vi "RVTBOX SampleCode.vi"(11 "Modbus TCP Setting":T1={"TCP address"="192.168.1.38", "CH"=enum."Port1", "Sample Rate"=7812, "Port"=502}) -> ()   [LabVIEW 2022 SP3]
uses:
  Ctl/Modbus Function TCP.ctl
  Ctl/TCP Setting.ctl
  DLL/Modbus.dll
panel:
  out "Waveform Chart":dbl[][](graph)=[[0.0015869140625, -0.000732421875, -0.001220703125], [0.0008544921875, -0.0009765625, 0.000244140625], [0.0006103515625, -0.001220703125, 0.001220703125], [0.0015869140625, -0.0006103515625, 0.00048828125], [0.001953125, 0.0, -0.00048828125], [0.0009765625, 0.0, -0.000732421875], [0.0010986328125, -0.000244140625, -0.0006103515625], [0.0020751953125, 0.000244140625, 0.0], [0.002197265625, 0.001220703125, 0.0006103515625], [0.0020751953125, 0.0009765625, -0.000244140625], [0.0020751953125, 0.0, -0.0018310546875], [0.0013427734375, 0.0, -0.001708984375], [0.00048828125, 0.0001220703125, -0.0008544921875], [0.0009765625, -0.000244140625, -0.0010986328125], [0.0009765625, -0.0008544921875, -0.00146484375], [-0.0003662109375, -0.0003662109375, -0.0003662109375], [-0.0010986328125, 0.0, 0.0001220703125], [-0.0003662109375, -0.000244140625, -0.0008544921875], [-0.0006103515625, -0.000244140625, -0.001708984375], [-0.00146484375, 0.0010986328125, 0.0], [-0.000732421875, 0.001953125, 0.002685546875], [0.000244140625, 0.0010986328125, 0.0037841796875], [0.0, 0.0003662109375, 0.002197265625], [-0.0006103515625, 0.0006103515625, -0.0006103515625]]
  out "Modbus Function":T2
  out "Failure  (Port1 ~ Port4)":bool[](array[boolean])
  out "Connted (Port1 ~ Port4)":bool[](array[boolean])
  out "Device ID":u16
  out "Stop Time":timestamp
  in  "stop":bool
  out "Data Length 抓資料後的剩餘長度":u16(graph)
  out "Iteration":i32
  out "Next #":u16
  out "error out":errorcluster
  # "BOX只能一次抓一個PORT 無法同時抓4個"
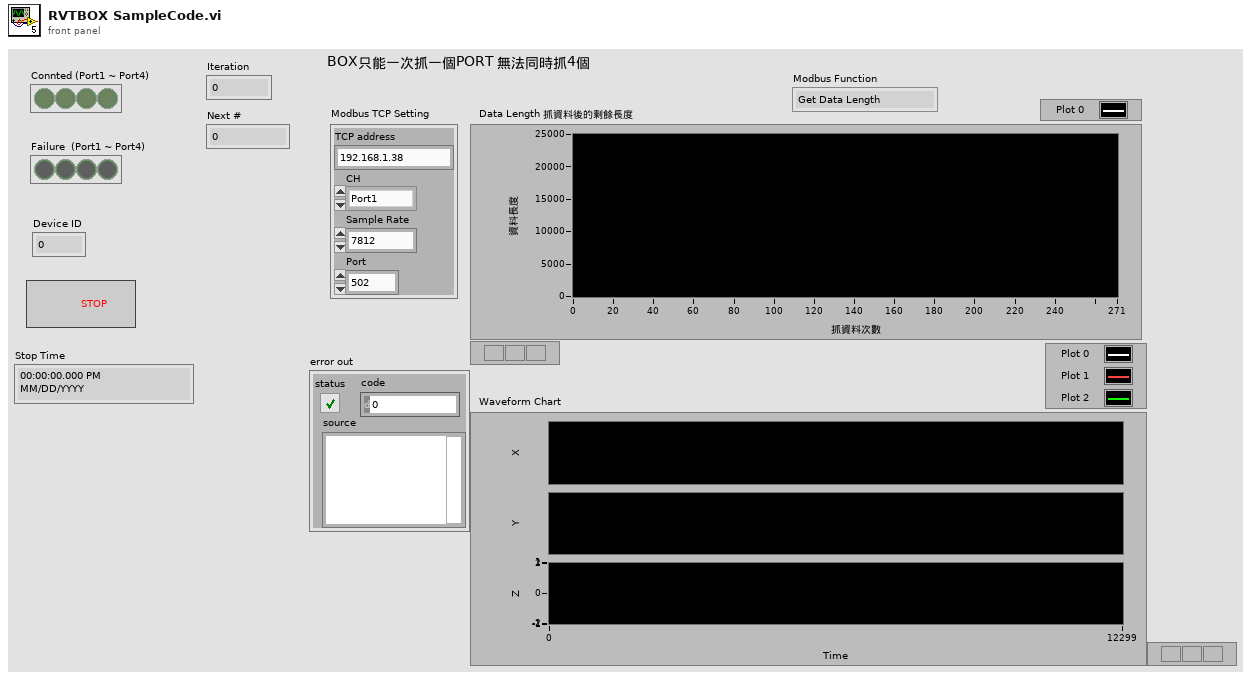
[diagram p1: front panel]
types:
  T1 = typedef "TCP Setting.ctl" = cluster{"TCP address":string, "CH":enum16{"Port1", "Port2", "Port3", "Port4"}, "Sample Rate":u16, "Port":i32}
  T2 = typedef "Modbus Function TCP.ctl" = enum16{"Get Data Length", "Normal Mode", "Bulk Mode", "Reconnect Port", "Recconect Box"}
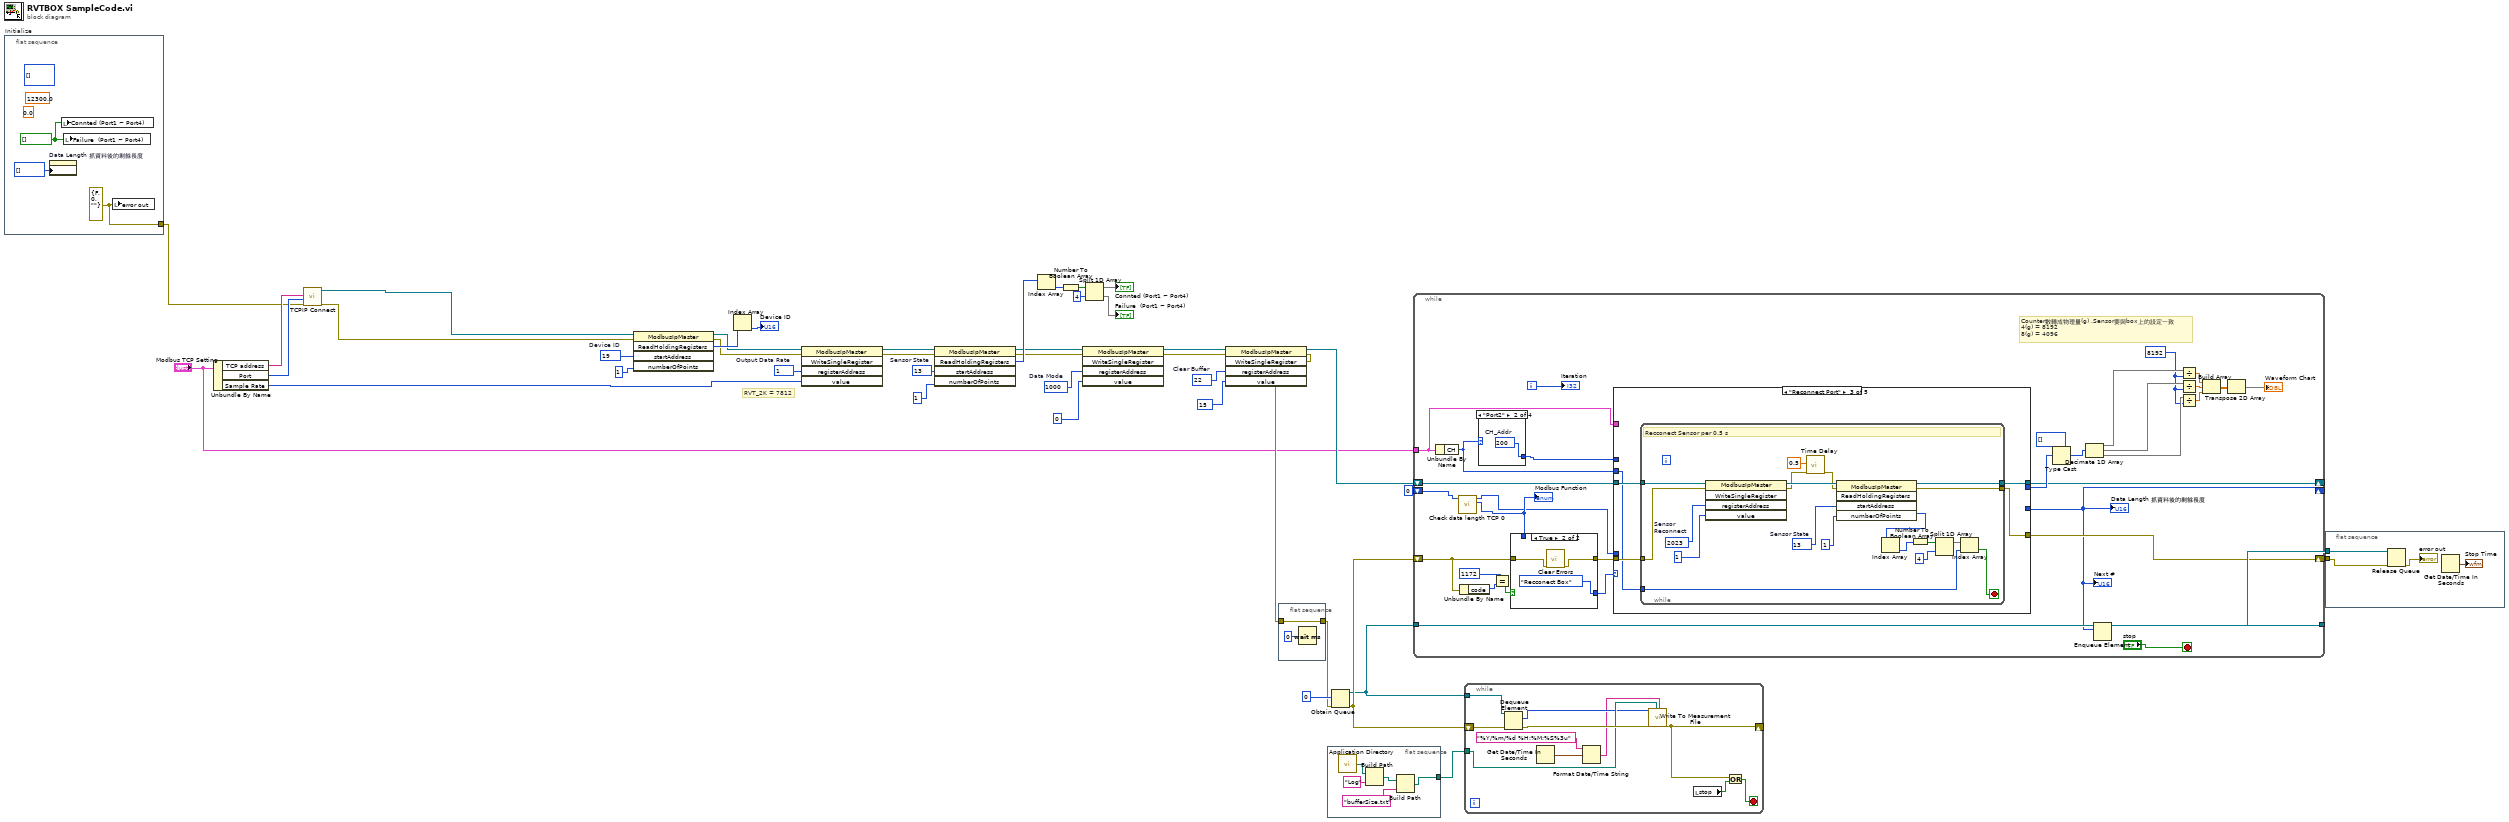
[diagram p0: block diagram]
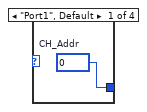
[diagram p3: hidden frame]
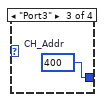
[diagram p4: hidden frame]
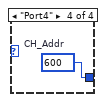
[diagram p5: hidden frame]
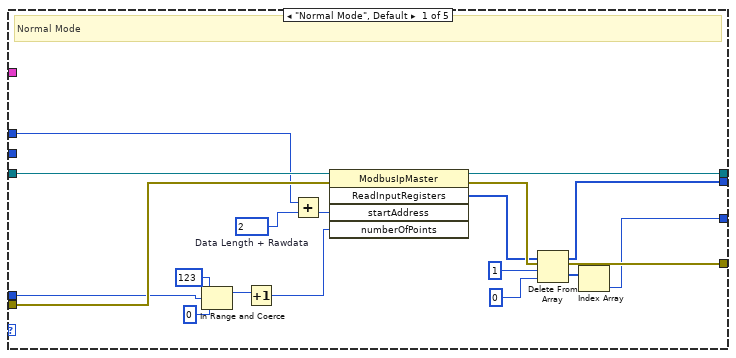
[diagram p6: hidden frame]
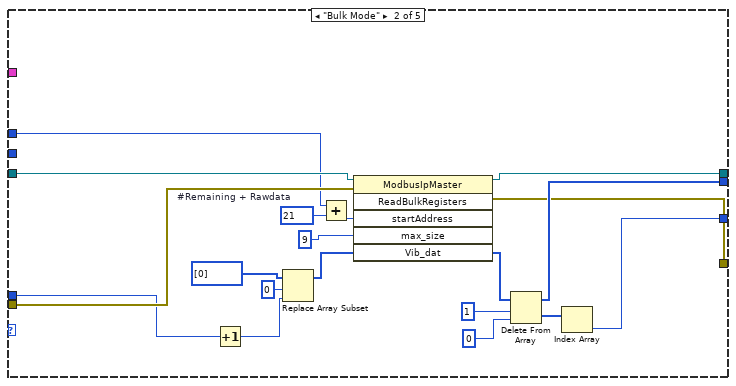
[diagram p7: hidden frame]
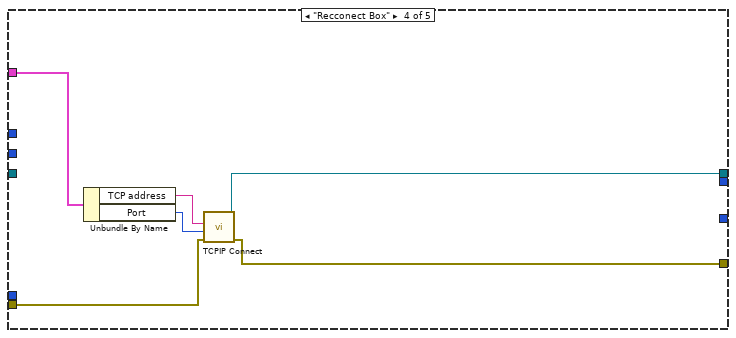
[diagram p8: hidden frame]
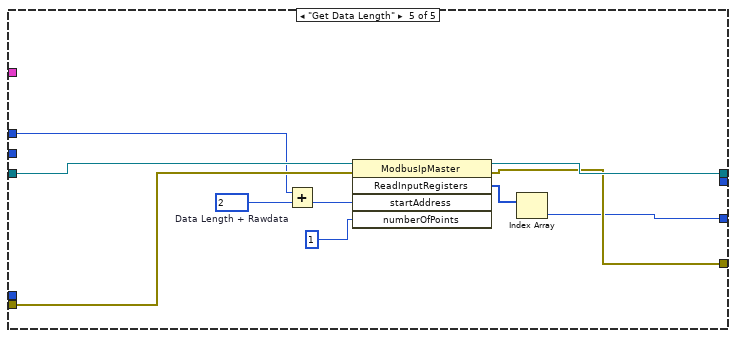
[diagram p9: hidden frame]
diagram:
  w14 = u16 1000  # Data Mode
  w17 = u16 22  # Clear Buffer
  w27 = u16 13  # Sensor State
  w32 = u16 19  # Device ID
  w34 = u16 1  # Output Data Rate
  # "RVT_2K = 7812"
  n1 = flat-sequence "Initialize" {
    tunnel: [w45] -> w7
    frame #0 {
      (unwired) 12300.0 ("X Scale.Range:Maximum")
      (unwired) 0.0 ("X Scale.Range:Minimum")
      (unwired) i16[][] []
      w44 = bool[] [] ("Failure ? (Port1 ~ Port4)")
      w45 = errorcluster {"status"=FALSE, "code"=0, "source"=""} ("error out")
      n2 = property on="Data Length 抓資料後的剩餘長度" class="WFChart (strict)"("History Data"=u16[] []) -> ()  [unwired: 2 in, 2 out]
      n3 = local write "Connted (Port1 ~ Port4)"(w44) -> ()
      n4 = local write "Failure  (Port1 ~ Port4)"(w44) -> ()
      n5 = local write "error out"(w45) -> ()
    }
  }
  n6 = Unbundle By Name("Modbus TCP Setting") -> ("TCP address"=w9:string, "Port"=w8:i32, "Sample Rate"=w11:u16)
  n7 = call "TCPIP Connect.vi"("error in (no error)"=w7, "Port"=w8, "TCP address"=w9) -> ("error out"=w1:errorcluster, "CreateIp"=w2:refnum<k24>)  [unwired: 7 in]
  n8 = invoke class="ModbusIpMaster" method="ReadHoldingRegisters"(reference=w2, error in=w1, "startAddress"=w32, "numberOfPoints"=u16 1) -> (reference out=w4:refnum<k24>, error out=w3:errorcluster, "ReadHoldingRegisters"=w31:u16[])  [unwired: 1 in, 2 out]
  n9 = Index Array(array=w31) -> (element=→"Device ID":u16)  [unwired: 1 in]
  n10 = invoke class="ModbusIpMaster" method="WriteSingleRegister"(reference=w4, error in=w3, "registerAddress"=w34, "value"=w11) -> (reference out=w25:refnum<k24>, error out=w24:errorcluster)  [unwired: 1 in, 3 out]
  n11 = invoke class="ModbusIpMaster" method="ReadHoldingRegisters"(reference=w25, error in=w24, "startAddress"=w27, "numberOfPoints"=u16 1) -> (reference out=w6:refnum<k24>, error out=w5:errorcluster, "ReadHoldingRegisters"=w23:u16[])  [unwired: 1 in, 2 out]
  n12 = Index Array(array=w23) -> (element=w22:u16)  [unwired: 1 in]
  n13 = Number To Boolean Array(number=w22) -> (Boolean array=w20:bool[])
  n14 = invoke class="ModbusIpMaster" method="WriteSingleRegister"(reference=w6, error in=w5, "registerAddress"=w14, "value"=u16 0) -> (reference out=w13:refnum<k24>, error out=w12:errorcluster)  [unwired: 1 in, 3 out]
  n15 = Split 1D Array(array=w20, index=4) -> (first subarray=→"Connted (Port1 ~ Port4)":bool[], second subarray=→"Failure  (Port1 ~ Port4)":bool[])
  n16 = invoke class="ModbusIpMaster" method="WriteSingleRegister"(reference=w13, error in=w12, "registerAddress"=w17, "value"=u16 15) -> (reference out=w28:refnum<k24>, error out=w29:errorcluster)  [unwired: 1 in, 3 out]
  n17 = flat-sequence {
    tunnel: w29 -> [w46]
    tunnel: [w46] -> w39
    frame #0 {
      n18 = Wait (ms)(milliseconds to wait=u32 0) -> ()  [unwired: 1 out]
    }
  }
  n19 = flat-sequence {
    tunnel: [w48] -> w35
    frame #0 {
      n20 = call <vilib>:"Application Directory.vi"() -> ("Application Directory"=w52:path)
      n21 = Build Path(base path=w52, name or relative path="Log") -> (appended path=w50:path)
      n22 = Build Path(base path=w50, name or relative path="bufferSize.txt") -> (appended path=w48:path)
    }
  }
  n23 = Obtain Queue(element data type=u16 0 ("Next # 2"), error in (no error)=w39) -> (queue out=w37:refnum<queue>, error out=w38:errorcluster)  [unwired: 3 in, 1 out]
  n24 = while {
    shift-right: [w79] -> w42
    shift-left: w38 -> [w68]
    shift-right: [w77] -> _
    shift-left: u16 0 ("# samples in buffer") -> [w64]
    shift-right: [w75] -> _
    shift-left: w28 -> [w84]
    tunnel: w37 -> [w78]
    tunnel: [w76] -> w36
    tunnel: "Modbus TCP Setting" -> [w65]
    i -> [w83]
    stop <- "stop" stop-if-true
    w58 = 8192 ("length")
    # "Counter數轉成物理量(g) ,Sensor要與box上的設定一致\n4(g) = 8192\n8(g) = 4096"
    n25 = Unbundle By Name(w65) -> ("CH"=w66:enum16{"Port1", "Port2", "Port3", "Port4"})
    n26 = call "Check data length TCP 0.vi"("# samples in buffer"=w64) -> ("Modbus Function"=w63:T2, "# samples in buffer out"=w62:u16)  [unwired: 9 in]
    "Modbus Function" <- w63
    n27 = Unbundle By Name(w68) -> ("code"=w72:i32)
    n28 = case shown="\"Port2\"" w66 {
      tunnel: [w90 w91 w92 w93] -> w74
      frame "Port1", Default {
        w90 = u16 0  # CH_Addr
      }
      frame "Port2" {
        w91 = u16 200  # CH_Addr
      }
      frame "Port3" {
        w92 = u16 400  # CH_Addr
      }
      frame "Port4" {
        w93 = u16 600  # CH_Addr
      }
    }
    n29 = Equal?(x=1172, y=w72) -> (x = y?=w70:bool)
    n30 = case shown="True" w70 {
      tunnel: [w85 Modbus_Function_TCP."Recconect Box" ("Modbus Function 2")] -> w69
      tunnel: w68 -> [w86 w89]
      tunnel: [w86 w88] -> w67
      tunnel: w63 -> [w85 _]
      frame False {
      }
      frame True {
        n31 = call <vilib>:"Clear Errors.vi"("error in (no error)"=w89) -> ("error out"=w88:errorcluster)  [unwired: 5 in, 1 out]
      }
    }
    n32 = case shown="\"Reconnect Port\"" w69 {
      tunnel: w84 -> [w99 w116 w135 _ w168]
      tunnel: [w101 w120 _ _ w164] -> w77
      tunnel: [w103 w118 w132 w156 w166] -> w79
      tunnel: [w100 w115 w131 w155 w167] -> w75
      tunnel: w67 -> [w104 w117 w134 w157 w169]
      tunnel: [w102 w119 _ _ _] -> w81
      tunnel: w62 -> [w96 w114 _ _ _]
      tunnel: w74 -> [w94 w112 _ _ w161]
      tunnel: w66 -> [_ _ w133 _ _]
      tunnel: w65 -> [_ _ _ w160 _]
      frame "Normal Mode", Default {
        w109 = u16 2  # Data Length + Rawdata
        # "Normal Mode"
        n33 = In Range and Coerce(upper limit=u16 123, x=w96, lower limit=u16 0) -> (coerced(x)=w105:u16)  [unwired: 1 out]
        n34 = Increment(x=w105) -> (x+1=w98:u16)
        n35 = Add(x=w94, y=w109) -> (x+y=w95:u16)
        n36 = invoke class="ModbusIpMaster" method="ReadInputRegisters"(reference=w99, error in=w104, "startAddress"=w95, "numberOfPoints"=w98) -> (reference out=w100:refnum<k24>, error out=w103:errorcluster, "ReadInputRegisters"=w97:u16[])  [unwired: 1 in, 2 out]
        n37 = Delete From Array(array=w97, length=1, index=0) -> (deleted portion=w108:u16[], array with subset deleted=w102:u16[])
        n38 = Index Array(array=w108) -> (element=w101:u16)  [unwired: 1 in]
      }
      frame "Bulk Mode" {
        w129 = u16 21  # #Remaining + Rawdata
        n39 = Increment(x=w114) -> (x+1=w123:u16)
        n40 = Replace Array Subset(array=u16[] [0], new element=w123, index=0) -> (w127:u16[])
        n41 = Add(x=w112, y=w129) -> (x+y=w113:u16)
        n42 = invoke class="ModbusIpMaster" method="ReadBulkRegisters"(reference=w116, error in=w117, "startAddress"=w113, "max_size"=i16 9, "Vib_dat"=w127) -> (reference out=w115:refnum<k24>, error out=w118:errorcluster, "Vib_dat"=w130:u16[])  [unwired: 1 in, 3 out]
        n43 = Delete From Array(array=w130, length=1, index=0) -> (deleted portion=w126:u16[], array with subset deleted=w119:u16[])
        n44 = Index Array(array=w126) -> (element=w120:u16)  [unwired: 1 in]
      }
      frame "Reconnect Port" {
        n45 = while {
          tunnel: w135 -> [w152]
          tunnel: w134 -> [w151]
          tunnel: w133 -> [w143]
          tunnel: [w140] -> w132
          tunnel: [w139] -> w131
          stop <- w142 stop-if-true
          w146 = u16 13  # Sensor State
          w154 = u16 2023  # Sensor  Reconnect
          # "Recconect Sensor per 0.5 s"
          n46 = invoke class="ModbusIpMaster" method="WriteSingleRegister"(reference=w152, error in=w151, "registerAddress"=w154, "value"=u16 1) -> (reference out=w144:refnum<k24>, error out=w137:errorcluster)  [unwired: 1 in, 3 out]
          n47 = call "Time Delay"("error in (no error)"=w137, "Delay Time (s)"=0.5) -> ("error out"=w136:errorcluster)  [unwired: 9 in]
          n48 = invoke class="ModbusIpMaster" method="ReadHoldingRegisters"(reference=w144, error in=w136, "startAddress"=w146, "numberOfPoints"=u16 1) -> (reference out=w139:refnum<k24>, error out=w140:errorcluster, "ReadHoldingRegisters"=w149:u16[])  [unwired: 1 in, 2 out]
          n49 = Index Array(array=w149) -> (element=w148:u16)  [unwired: 1 in]
          n50 = Number To Boolean Array(number=w148) -> (Boolean array=w147:bool[])
          n51 = Split 1D Array(array=w147, index=4) -> (first subarray=w150:bool[])  [unwired: 1 out]
          n52 = Index Array(array=w150, index=w143) -> (element=w142:bool)
        }
      }
      frame "Recconect Box" {
        n53 = Unbundle By Name(w160) -> ("TCP address"=w159:string, "Port"=w158:i32)
        n54 = call "TCPIP Connect.vi"("error in (no error)"=w157, "Port"=w158, "TCP address"=w159) -> ("error out"=w156:errorcluster, "CreateIp"=w155:refnum<k24>)  [unwired: 7 in]
      }
      frame "Get Data Length" {
        w170 = u16 2  # Data Length + Rawdata
        n55 = Add(x=w161, y=w170) -> (x+y=w162:u16)
        n56 = invoke class="ModbusIpMaster" method="ReadInputRegisters"(reference=w168, error in=w169, "startAddress"=w162, "numberOfPoints"=u16 1) -> (reference out=w167:refnum<k24>, error out=w166:errorcluster, "ReadInputRegisters"=w165:u16[])  [unwired: 1 in, 2 out]
        n57 = Index Array(array=w165) -> (element=w164:u16)  [unwired: 1 in]
      }
    }
    "Next #" <- w77
    "Data Length 抓資料後的剩餘長度" <- w77
    n58 = Type Cast(type=i16[] [], x=w81) -> (*(type *) &x=w80:i16[])
    n59 = Decimate 1D Array(w80) -> (w61:i16[], w60:i16[], w59:i16[])
    n60 = Enqueue Element(queue=w78, element=w77) -> (queue out=w76:refnum<queue>)  [unwired: 2 in, 2 out]
    n61 = Divide(x=w61, y=w58) -> (x/y=w57:dbl[])
    n62 = Divide(x=w60, y=w58) -> (x/y=w56:dbl[])
    n63 = Divide(x=w59, y=w58) -> (x/y=w55:dbl[])
    n64 = Build Array(w57, w56, w55) -> (w54:dbl[][])
    n65 = Transpose 2D Array(2D array=w54) -> (transposed array=→"Waveform Chart":dbl[][])
    "Iteration" <- w83
  }
  n66 = while {
    tunnel: w37 -> [w180]
    shift-right: [w176] -> _
    shift-left: w38 -> [w181]
    tunnel: w35 -> [w175]
    stop <- w178 stop-if-true
    n67 = Dequeue Element(queue=w180, error in (no error)=w181) -> (element=w174:u16, error out=w177:errorcluster)  [unwired: 1 in, 2 out]
    n68 = Get Date/Time In Seconds() -> (seconds since 1Jan1904=w173:timestamp)
    n69 = Format Date/Time String(time format string (%c)="%Y/%m/%d %H:%M:%S%3u", seconds (now)=w173) -> (date/time string=w172:string)  [unwired: 1 in]
    n70 = call "Write To Measurement File"("Signals"=w174, "error in (no error)"=w177, "Filename"=w175, "Comment"=w172) -> ("error out"=w176:errorcluster)  [unwired: 13 in, 2 out]
    n71 = local read "stop"() -> (w179:bool)
    n72 = Or(x=w176, y=w179) -> (x .or. y?=w178:bool)
  }
  n73 = flat-sequence {
    tunnel: w42 -> [w184]
    tunnel: w36 -> [w182]
    frame #0 {
      n74 = Release Queue(queue=w182, error in (no error)=w184) -> (error out=→"error out":errorcluster)  [unwired: 1 in, 2 out]
      n75 = Get Date/Time In Seconds() -> (seconds since 1Jan1904=→"Stop Time":timestamp)
    }
  }
